vi "Cleanup.vi"(8 "error in (no error)":errorcluster, 11 "Start Bug Remover in":refnum<class "Start Bug Remover.lvclass">) -> (0 "error out":errorcluster, 3 "Start Bug Remover out":refnum<class "Start Bug Remover.lvclass">)   [LabVIEW 2019, in "Start Bug Remover.lvclass"]
uses:
  <vilib>/gpm_packages/@cs/Car-wash/Source/Process Steps/Start Bug Remover/Start Bug Remover.lvclass
  <vilib>/gpm_packages/@cs/Car-wash/Source/iProcess Step Model/iProcess Step Model/iProcess Step Model.lvclass
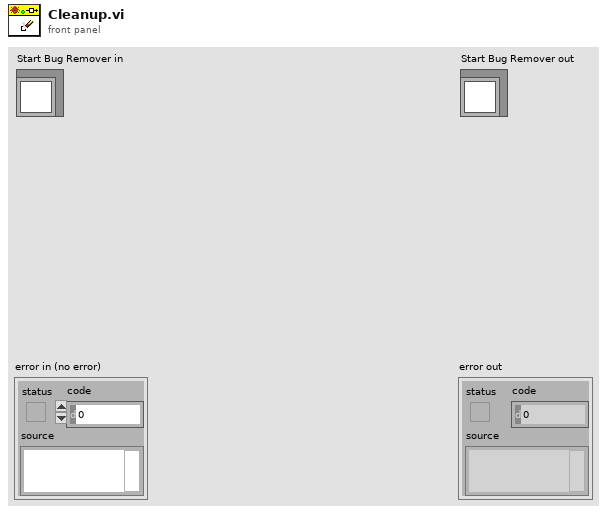
[diagram p1: front panel]
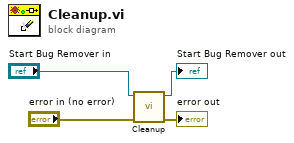
[diagram p0: block diagram]
diagram:
  n1 = call-parent "Cleanup.vi"("error in (no error)"="error in (no error)", "iProcess Step Model in"="Start Bug Remover in") -> ("error out"=→"error out":errorcluster, "iProcess Step Model out"=→"Start Bug Remover out":refnum<class "Start Bug Remover.lvclass">)  [unwired: 8 in]
